vi "FFT Co-processor (FPGA).vi"() -> ()   [LabVIEW 2014]
doc: "Data From Host Loop:\nThe FPGA target recieves a signal from the host from the Host-to-FPGA DMA FIFO and stores that data in the FIFO IN target-scoped FIFO. FIFO IN will not be written to if there is no information being read from the host and the Host-to-FPGA FIFO has timed out. The loop will stop if the user presses the stop control button or if the FIFO IN times out and data transfer from the host to the target is complete.\n\nFFT Processing Loop:\nWhen the FFT Express VI has signaled that it is ready for input, it will begin to read data from the FIFO IN target-scoped FIFO. The user has control over the output of the FFT Express VI. As the FFT VI computes the FFT it writes the resulting data to the FIFO OUT target-scoped VI when the FFT output is valid. The loop will stop if the user presses the stop control button or if the FIFO OUT times out and data transfer from the FFT VI to the FIFO is complete.\n\nData To Host Loop:\nFIFO OUT transfers data back to the host by writing the computed FFT signal data to the FPGA-to-Host DMA FIFO. When there is no data in FIFO OUT, it times out and stops writing to the host. At this point the data transfer is complete."
uses:
  <vilib>/Platform/TimedLoop/XDataNode/timing_clust.ctl
  <vilib>/Platform/TimedLoop/XDataNode/nitl_modes.ctl
  <vilib>/Platform/TimedLoop/XDataNode/wakeup.ctl
  <vilib>/rvi/Analysis/measure/FFT/simModelSupport/niFPGA FFT Streaming Sim Properties.ctl
  <vilib>/rvi/Analysis/measure/FFT/simModelSupport/niFPGA FFT Sim Stream Group Properties.ctl
  <vilib>/rvi/Analysis/measure/FFT/simModelSupport/niFPGA FFT Sim Types.ctl
  <vilib>/rvi/Analysis/measure/FFT/simModelSupport/niFpgaFFTSimArithmeticProperties.ctl
  <vilib>/rvi/Analysis/measure/FFT/simModelSupport/niFpgaFFTSimDfxp.ctl
  <vilib>/fxp/LVFixedPointQuantizationPolicyTypeDef.ctl
  <vilib>/rvi/Analysis/measure/FFT/XNode/niFpgaFFTButterflyDelays.ctl
  <vilib>/rvi/Emulation/niFpgaSctlEmulationGetInTimedLoop.vi
  <vilib>/rvi/Emulation/niFpgaEmulationReportErrorSimple.vi
  <vilib>/rvi/Emulation/niFpgaGetClockAttributes.vi
  <vilib>/rvi/Emulation/niFpgaCriticalErrorInLSC.vi
  <vilib>/rvi/Emulation/niFpgaProcessEmulError.vi
  <vilib>/rvi/Emulation/niFpgaEmulationIsFPGAContextNoSignature.vi
  <vilib>/rvi/errors/niFpgaSetErrorForExecOnDevCompSimple.vi
  <vilib>/rvi/eio/common/nirviEmuReportErrorAndStop.vi
  <vilib>/rvi/DataTransferAndStorage/Container/Common/niFpgaContainerGetUniqueNameForEmu.vi
  <vilib>/rvi/FIFO/Fifo_Resource/nirvififoEmulationSetSize.vi
  <vilib>/rvi/FIFO/Fifo_Resource/nirviFifoEmulationQueueMgr.vi
  <instcachedir>/0/nirviFifoEmulationQueueMgr_E5CAEC123FF24DC58D834DCA3CDAA9B5.lvgen/nirviFifoEmulationQueueMgr_E5CAEC123FF24DC58D834DCA3CDAA9B5_002.vi
  <vilib>/Utility/error.llb/Clear Errors.vi
  <vilib>/rvi/FIFO/Fifo_Resource/nirvififoEmulationCreateLock.vi
  <vilib>/rvi/FIFO/Fifo_Resource/nirvififoEmulationObtainLock.vi
  <vilib>/rvi/FIFO/Fifo_Resource/nirvififoEmulationReleaseLock.vi
  <vilib>/rvi/occurrence/nirviWaitOnOccurrenceBase.vi
  <vilib>/rvi/errors/nirviReportUnexpectedCaseInternalError.vi
  <vilib>/rvi/errors/nirviReportUnexpectedCaseInternalError (U32).vi
  <vilib>/rvi/Analysis/measure/FFT/simModelSupport/niFpgaFFTSimModelStreamingCore.vi
  <vilib>/rvi/FIFO/Fifo_Resource/nirvififoEmulationDetermineInputValidOut.vi
  <vilib>/rvi/interface/RandomDataEmulation/niFpgaRandomDataHandleErrors.vi
  <vilib>/Platform/TimedLoop/XDataNode/XDataNode.xnode
  <vilib>/rvi/DataTransferAndStorage/Container/XNode/niFpgaContainer.xnode
  <vilib>/rvi/FIFO/Fifo_Resource/nirvififoEmulationRead.vi
  <vilib>/rvi/Analysis/measure/FFT/XNode/niFpgaFFT.xnode
  <vilib>/rvi/FIFO/Fifo_Resource/nirvififoEmulationWrite.vi
  <vilib>/rvi/interface/RandomDataEmulation/nirviRandomDataFpgaReadWriteTemplate.vi
  <vilib>/Platform/TimedLoop/XDataNode/XDNodeRunTimeDep.lvlib
panel:
  in  "FFT Size":i16=8
  out "FFT Out":i32
  out "FIFO In (loop 2)":i32
  out "FIFO In":i32
  out "Host to FPGA":i32
  in  "stop":bool
  # "This FPGA VI continuously receives data from the host, performs a 1 kByte FFT, and then transfers the FFT results back to the host.  The input data type for the FFT is a 16-bit fixed point number with 8 bits of integer precision."
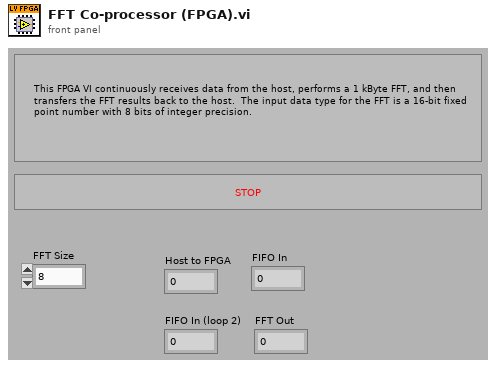
[diagram p1: front panel]
types:
  T1 = typedef "XDNodeRunTimeDep.lvlib/timing_clust.ctl" = cluster{"Expected End [f-1]":u64, "Actual End [f-1]":u64, "Finished Late? [f-1]":bool, "Expected End [i-1]":u64, "Actual End [i-1]":u64, "Finished Late? [i-1]":bool, "Expected Start [i]":u64, "Actual Start [i]":u64, "Expected Start [f]":u64, "Actual Start [f]":u64, "Source Name":string, "Structure Name":string, "Period":i64, "Deadline":i64, "Offset":i64, "Start":i64, "Priority":i32, "Timeout":i32, "Mode":T2, "Wakeup Reason":T3, "Error":errorcluster, "Source Type":string, "Secondary Source Type":string, "Global End Time":u64, "Global Start Time":u64, "Frame Duration":u64, "Iteration Duration":u64, "Assigned CPU":i32, "I/O Scan Engine Mode":u32}
  T2 = typedef "XDNodeRunTimeDep.lvlib/nitl_modes.ctl" = enum32{"No Change", "Process missed periods, maintain original phase", "Discard missed periods, maintain original phase", "Process missed periods, ignore original phase", "Discard missed periods, ignore original phase"}
  T3 = typedef "XDNodeRunTimeDep.lvlib/wakeup.ctl" = enum32{"Normal", "Aborted", "Asynchronous wakeup", "Timing source error", "Timed loop error", "Timeout"}
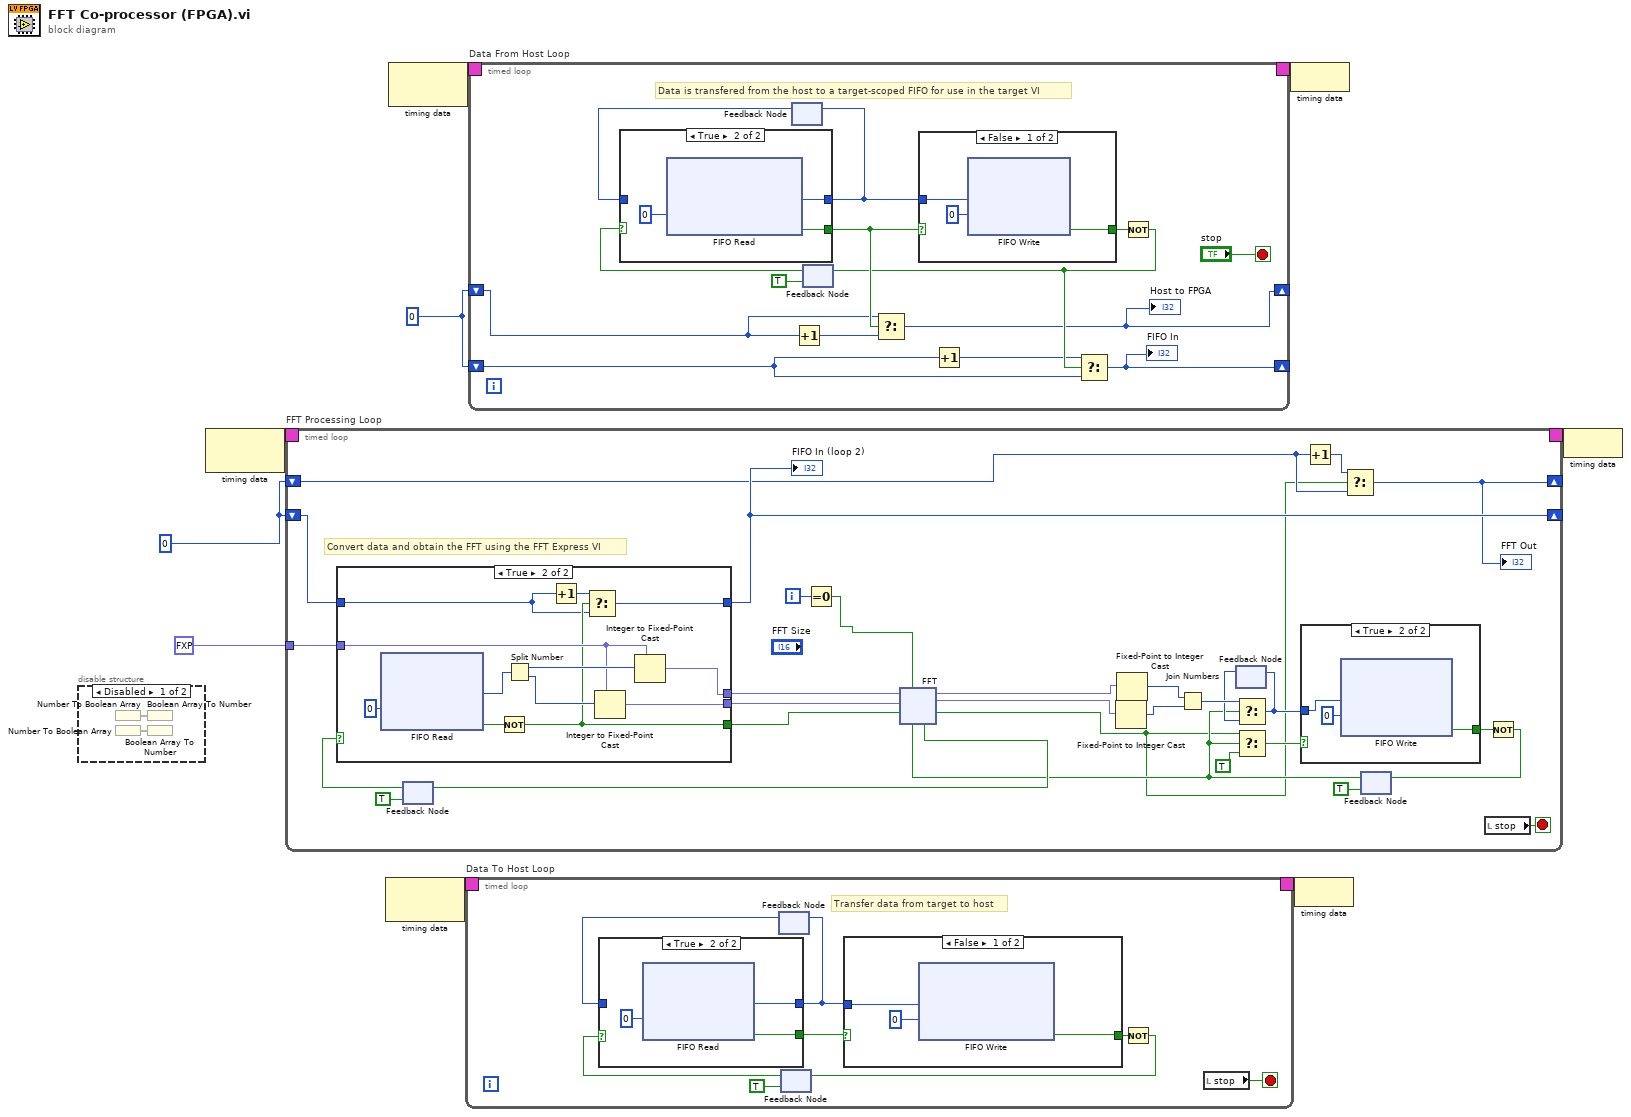
[diagram p0: block diagram]
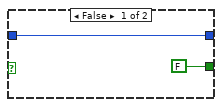
[diagram p3: hidden frame]
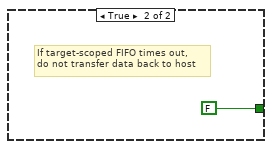
[diagram p4: hidden frame]
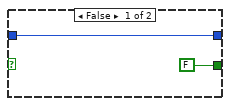
[diagram p5: hidden frame]
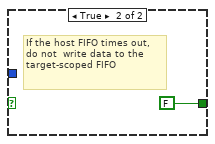
[diagram p6: hidden frame]
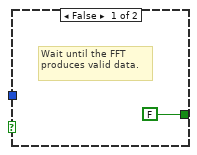
[diagram p7: hidden frame]
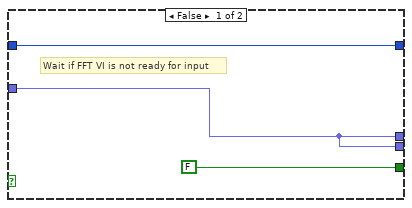
[diagram p8: hidden frame]
diagram:
  w1 = 0 ("Timeout")
  w2 = 0 ("Timeout")
  n1 = disable-structure shown="Disabled" {
    frame Disabled {
      n2 = Number To Boolean Array() -> (Boolean array=w11:bool[])  [unwired: 1 in]
      n3 = Number To Boolean Array() -> (Boolean array=w10:bool[])  [unwired: 1 in]
      n4 = Boolean Array To Number(Boolean array=w11) -> ()  [unwired: 1 out]
      n5 = Boolean Array To Number(Boolean array=w10) -> ()  [unwired: 1 out]
    }
    frame Enabled {
    }
  }
  n6 = node-c288() -> (w9:T1)  [unwired: 1 out]
  n7 = timed-loop "FFT Processing Loop" {
    timing: w9 -> [_]
    timing-out: [_] -> w8
    tunnel: fxp<+/-,24,4> 0.0 ("real data in") -> [w24]
    shift-right: [w22] -> _
    shift-left: w1 -> [w23]
    shift-right: [w19] -> _
    shift-left: w1 -> [w20]
    i -> [w38]
    stop <- w35 stop-if-true
    # "Convert data and obtain the FFT using the FFT Express VI"
    n8 = feedback #1(TRUE ("ready for data")) -> (w40:bool)
    n9 = case shown="True" w40 {
      tunnel: [FALSE w77] -> w25
      tunnel: [w72 w80] -> w17
      tunnel: w24 -> [w72 w79]
      tunnel: [w72 w78] -> w16
      tunnel: w23 -> [w71 w75]
      tunnel: [w71 w74] -> w22
      frame False {
        # "Wait if FFT VI is not ready for input"
      }
      frame True {
        n10 = xnode ("FIFO Read")("Timeout"=0) -> ("Element"=w83:u64, "Timed Out?"=w85:bool)  [unwired: 1 in, 1 out]
        n11 = Not(x=w85) -> (.not. x?=w77:bool)
        n12 = Split Number(x=w83) -> (hi(x)=w82:u32, lo(x)=w81:u32)
        n13 = Increment(x=w75) -> (x+1=w76:i32)
        n14 = Select(t=w76, s=w77, f=w75) -> (s? t:f=w74:i32)
        n15 = Integer to Fixed-Point Cast(fixed-point type=w79, integer=w81) -> (fixed-point=w78:fxp<+/-,24,4>)
        n16 = Integer to Fixed-Point Cast(fixed-point type=w79, integer=w82) -> (fixed-point=w80:fxp<+/-,24,4>)
      }
    }
    "FIFO In (loop 2)" <- w22
    n17 = Equal To 0?(x=w38) -> (x = 0?=w37:bool)
    n18 = feedback #2() -> (w30:u64)  [unwired: 1 out]
    n19 = Increment(x=w20) -> (x+1=w21:i32)
    n20 = feedback #3(TRUE ("ready for data")) -> (w27:bool)
    n21 = xnode "FFT"("real data in"=w17, "reset"=w37, "imaginary data in"=w16, "input valid"=w25, "ready for output"=w27) -> ("ready for input"=w36:bool, "real data out"=w15:fxp<+/-,28,8>, "imaginary data out"=w14:fxp<+/-,28,8>, "output valid"=w18:bool)  [unwired: 1 out]
    n22 = feedback-in #1(w36) -> ()
    n23 = Fixed-Point to Integer Cast(1:w14) -> (0:w13:i32)
    n24 = Fixed-Point to Integer Cast(1:w15) -> (0:w12:i32)
    n25 = Join Numbers(hi=w12, lo=w13) -> ((hi.lo)=w31:u64)
    n26 = Select(t=w31, s=w27, f=w30) -> (s? t:f=w29:u64)
    n27 = feedback-in #2(w29) -> ()
    n28 = Select(t=w18, s=w27, f=TRUE) -> (s? t:f=w28:bool)
    n29 = case shown="True" w28 {
      tunnel: [FALSE ("Timed Out?") w69] -> w34
      tunnel: w29 -> [_ w68]
      frame False {
        # "Wait until the FFT produces valid data."
      }
      frame True {
        n30 = xnode ("FIFO Write")("Element"=w68, "Timeout"=0) -> ("Timed Out?"=w69:bool)  [unwired: 1 in, 1 out]
      }
    }
    n31 = Select(t=w21, s=w18, f=w20) -> (s? t:f=w19:i32)
    "FFT Out" <- w19
    n32 = local read "stop"() -> (w35:bool)
    n33 = Not(x=w34) -> (.not. x?=w32:bool)
    n34 = feedback-in #3(w32) -> ()
  }
  n35 = node-c288() -> (w5:T1)  [unwired: 1 out]
  n36 = node-c288() -> (w7:T1)  [unwired: 1 out]
  n37 = timed-loop "Data To Host Loop" {
    timing: w5 -> [_]
    timing-out: [_] -> w4
    stop <- w94 stop-if-true
    # "Transfer data from target to host"
    n38 = feedback #4() -> (w92:u64)  [unwired: 1 out]
    n39 = feedback #5(TRUE) -> (w88:bool)
    n40 = case shown="True" w88 {
      tunnel: [FALSE ("Timed Out?") w99] -> w95
      tunnel: [w97 w98] -> w93
      tunnel: w92 -> [w97 _]
      frame False {
      }
      frame True {
        n41 = xnode ("FIFO Read")("Timeout"=0) -> ("Element"=w98:u64, "Timed Out?"=w99:bool)  [unwired: 1 in, 1 out]
      }
    }
    n42 = feedback-in #4(w93) -> ()
    n43 = case shown="False" w95 {
      tunnel: [w101 FALSE ("Timed Out?")] -> w91
      tunnel: w93 -> [w103 _]
      frame False {
        n44 = xnode ("FIFO Write")("Element"=w103, "Timeout"=0) -> ("Timed Out?"=w101:bool)  [unwired: 1 in, 1 out]
      }
      frame True {
        # "If target-scoped FIFO times out, \ndo not transfer data back to host"
      }
    }
    n45 = Not(x=w91) -> (.not. x?=w89:bool)
    n46 = feedback-in #5(w89) -> ()
    n47 = local read "stop"() -> (w94:bool)
  }
  n48 = timed-loop "Data From Host Loop" {
    timing: w7 -> [_]
    timing-out: [_] -> w6
    shift-right: [w112] -> _
    shift-left: w2 -> [w110]
    shift-right: [w111] -> _
    shift-left: w2 -> [w108]
    stop <- "stop" stop-if-true
    # "Data is transfered from the host to a target-scoped FIFO for use in the target VI"
    n49 = feedback #6() -> (w115:u64)  [unwired: 1 out]
    n50 = Increment(x=w110) -> (x+1=w109:i32)
    n51 = feedback #7(TRUE) -> (w117:bool)
    n52 = case shown="True" w117 {
      tunnel: [FALSE ("Timed Out?") w125] -> w114
      tunnel: [w122 w123] -> w116
      tunnel: w115 -> [w122 _]
      frame False {
      }
      frame True {
        n53 = xnode ("FIFO Read")("Timeout"=0) -> ("Element"=w123:u64, "Timed Out?"=w125:bool)  [unwired: 1 in, 1 out]
      }
    }
    n54 = feedback-in #6(w116) -> ()
    n55 = Select(t=w110, s=w114, f=w109) -> (s? t:f=w112:i32)
    "Host to FPGA" <- w112
    n56 = case shown="False" w114 {
      tunnel: w116 -> [w127 _]
      tunnel: [w126 FALSE ("Timed Out?")] -> w119
      frame False {
        n57 = xnode ("FIFO Write")("Element"=w127, "Timeout"=0) -> ("Timed Out?"=w126:bool)  [unwired: 1 in, 1 out]
      }
      frame True {
        # "If the host FIFO times out, do not  write data to the target-scoped FIFO"
      }
    }
    n58 = Increment(x=w108) -> (x+1=w107:i32)
    n59 = Not(x=w119) -> (.not. x?=w113:bool)
    n60 = feedback-in #7(w113) -> ()
    n61 = Select(t=w107, s=w113, f=w108) -> (s? t:f=w111:i32)
    "FIFO In" <- w111
  }
  n62 = node-c288(w6) -> ()
  n63 = node-c288(w4) -> ()
  n64 = node-c288(w8) -> ()
